vi "GetInnerTunnels.vi"(6 "error in":errorcluster, 9 "FlatSequenceFrame in":refnum<class "FlatSequenceFrame.lvclass">) -> (0 "error out":errorcluster, 3 "FlatSequenceFrame out":refnum<class "FlatSequenceFrame.lvclass">, 4 "right inside":i32[](array[numeric]), 5 "left inside":i32[](array[numeric]))   [LabVIEW 2014, in "FlatSequenceFrame.lvclass"]
uses:
  FlatSequenceFrame.lvclass
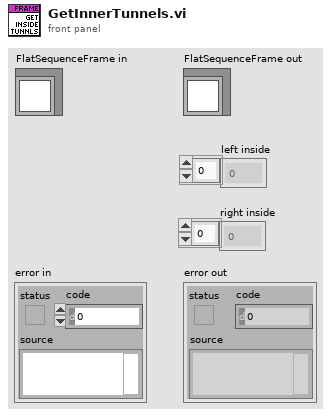
[diagram p1: front panel]
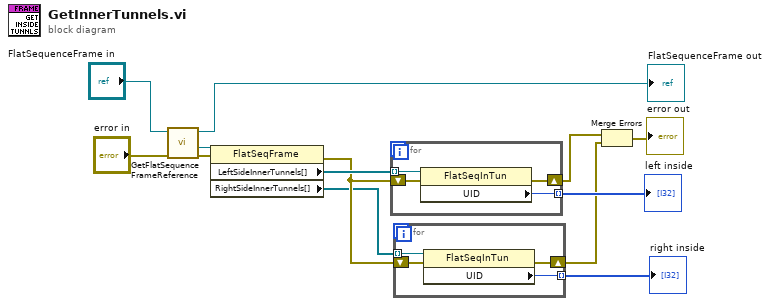
[diagram p0: block diagram]
diagram:
  n1 = call "GetFlatSequenceFrameReference.vi"("error in"="error in", "FlatSequence in"="FlatSequenceFrame in") -> ("error out"=w10:errorcluster, "reference out"=w11:refnum<vi>, "FlatSequence out"=→"FlatSequenceFrame out":refnum<class "FlatSequenceFrame.lvclass">)  [unwired: 7 in]
  n2 = property class="FlatSeqFrame"(reference=w11, error in=w10) -> (error out=w6:errorcluster, "LeftSideInnerTunnels[]"=w8:refnum<vi>[], "RightSideInnerTunnels[]"=w5:refnum<vi>[])  [unwired: 1 out]
  n3 = for {
    tunnel: w8 -> [w17] mode=indexing
    shift-right: [w15] -> w1
    shift-left: w6 -> [w16]
    tunnel: [w14] -> w7 mode=indexing
    n4 = property class="FlatSeqInTun"(reference=w17, error in=w16) -> (error out=w15:errorcluster, "UID"=w14:i32)  [unwired: 1 out]
  }
  "left inside" <- w7
  n5 = for {
    tunnel: w5 -> [w21] mode=indexing
    shift-right: [w19] -> w2
    shift-left: w6 -> [w20]
    tunnel: [w18] -> w4 mode=indexing
    n6 = property class="FlatSeqInTun"(reference=w21, error in=w20) -> (error out=w19:errorcluster, "UID"=w18:i32)  [unwired: 1 out]
  }
  "right inside" <- w4
  n7 = Merge Errors(w1, w2) -> (→"error out":errorcluster)
